vi "HEWH Gas Thermal Stabilization Check.vi"(6 "RTDOut-RTDin Delta":dbl[](array[numeric]), 9 "RTDout":dbl[](array[numeric]), 10 "RTDout-RTDin Current":dbl, 11 "Target RTDout-RTDin":dbl) -> (3 "Gas Thermal Stabilization Complete":bool)   [LabVIEW 2019]
panel:
  out "error out":errorcluster
  in  "error in (no error)":errorcluster
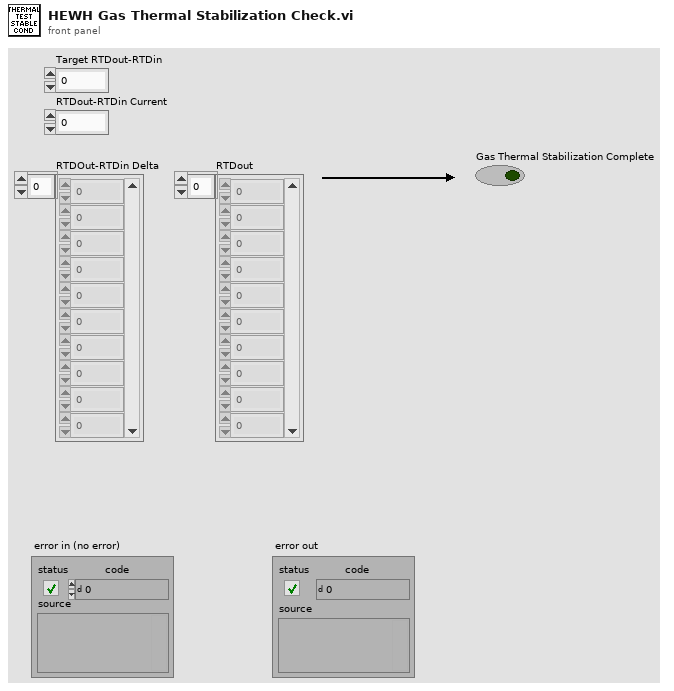
[diagram p1: front panel]
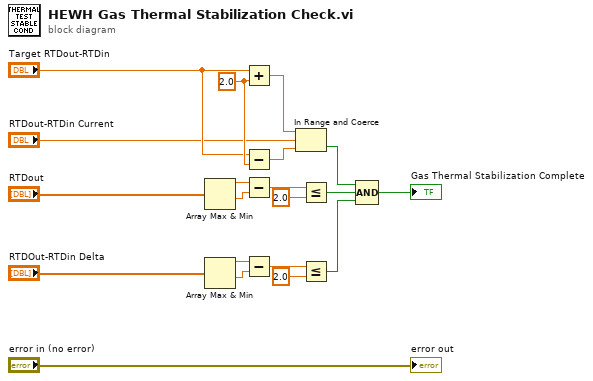
[diagram p0: block diagram]
diagram:
  w18 = 2.0 ("y")
  n1 = Array Max & Min(array="RTDout") -> (max value=w3:dbl, min value=w4:dbl)  [unwired: 2 out]
  n2 = Array Max & Min(array="RTDOut-RTDin Delta") -> (max value=w10:dbl, min value=w9:dbl)  [unwired: 2 out]
  n3 = Add(x="Target RTDout-RTDin", y=w18) -> (x+y=w16:dbl)
  n4 = Subtract(x="Target RTDout-RTDin", y=w18) -> (x-y=w19:dbl)
  n5 = Subtract(x=w3, y=w4) -> (x-y=w5:dbl)
  n6 = Subtract(x=w10, y=w9) -> (x-y=w8:dbl)
  n7 = In Range and Coerce(upper limit=w16, x="RTDout-RTDin Current", lower limit=w19) -> (In Range?=w20:bool)  [unwired: 1 out]
  n8 = Less Or Equal?(x=w5, y=2.0) -> (x <= y?=w12:bool)
  n9 = Less Or Equal?(x=w8, y=2.0) -> (x <= y?=w13:bool)
  n10 = Compound Arithmetic op=AND(w20, w12, w13) -> (→"Gas Thermal Stabilization Complete":bool)
  "error out" <- "error in (no error)"
